vi "Add Core Dependencies.vi"(8 "error in (no error)":errorcluster, 11 "Item Ref in":T1 format="%.0x") -> (0 "error out":errorcluster, 3 "Device Ref out":T1 format="%.0x")   [LabVIEW 2017, in "DSF System Explorer.lvlib"]
uses:
  DSF System Explorer.lvlib
  <vilib>/NI Veristand/Custom Device API/Custom Device Item Ref.ctl
  <vilib>/NI Veristand/Custom Device API/Custom Device File Dependency.ctl
  <vilib>/NI Veristand/Custom Device API/Path Specification.ctl
  <vilib>/NI Veristand/Custom Device API/Path Type.ctl
  <vilib>/NI Veristand/Custom Device API/Custom Device Supported Target.ctl
  <vilib>/NI Veristand/Custom Device API/Custom Device API.lvlib
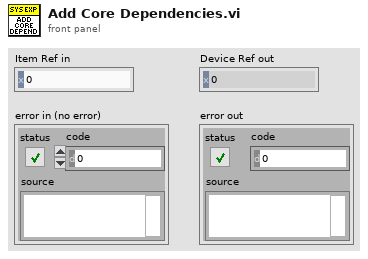
[diagram p1: front panel]
types:
  T1 = typedef "Custom Device API.lvlib/Custom Device Item Ref.ctl" = u64
  T2 = typedef "Custom Device API.lvlib/Custom Device Target Type.ctl" = enum16{"PharLap", "VxWorks", "Windows", "Linux_32_ARM", "Linux_x64"}
  T3 = typedef "Custom Device API.lvlib/Custom Device Supported Target.ctl" = enum16{"All", "PharLap", "VxWorks", "Windows", "Linux_32_ARM", "Linux_x64", "PharLap & Windows", "PharLap & VxWorks", "VxWorks & Windows"}
  T4 = typedef "Custom Device API.lvlib/Path Type.ctl" = enum16{"Absolute", "To Base", "To Common Data Dir", "To Application Data Dir"}
  T5 = typedef "Custom Device API.lvlib/Custom Device File Dependency.ctl" = cluster{"Source":T6, "RT Destination":path, "ForceDownload?":bool, "SupportedTarget":T3, "Version":string}
  T6 = typedef "Custom Device API.lvlib/Path Specification.ctl" = cluster{"Path":path, "Type":T4}
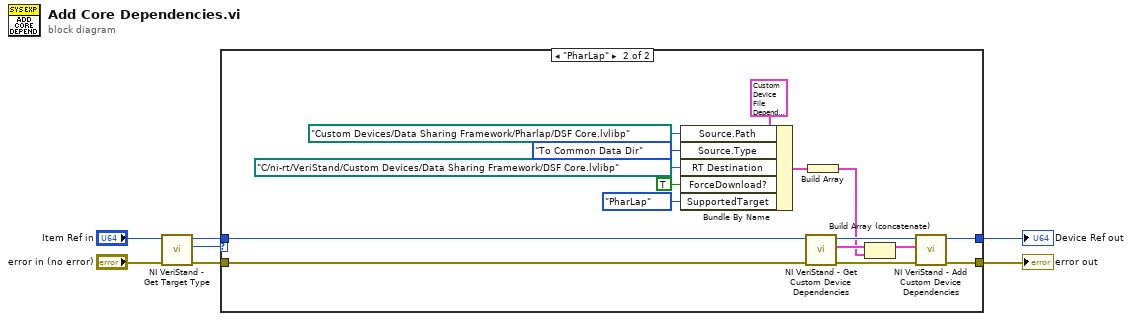
[diagram p0: block diagram]
diagram:
  n1 = call <vilib>:"NI VeriStand - Get Target Type.vi"("error in (no error)"="error in (no error)", "Item Ref in"="Item Ref in") -> ("error out"=w6:errorcluster, "Target Type"=w7:T2, "Item Ref out"=w5:T1)  [unwired: 7 in]
  n2 = case shown="\"PharLap\"" w7 {
    tunnel: [w9 w12] -> w1
    tunnel: [w8 w11] -> w2
    tunnel: w5 -> [w8 w13]
    tunnel: w6 -> [w9 w14]
    frame "Windows", Default {
      # "Don't add dependency for Windows or unsupported target type."
    }
    frame "PharLap" {
      n3 = Bundle By Name(cluster=T5 {"Source"={"Path"=path "", "Type"=enum."Absolute"}, "RT Destination"=path "", "ForceDownload?"=FALSE, "SupportedTarget"=enum."PharLap", "Version"=""} ("Dependencies"), "Source.Path"=path "Custom Devices/Data Sharing Framework/Pharlap/DSF Core.lvlibp", "Source.Type"=Path_Type."To Common Data Dir", "RT Destination"=path "C:/ni-rt/VeriStand/Custom Devices/Data Sharing Framework/DSF Core.lvlibp", "ForceDownload?"=TRUE, "SupportedTarget"=Custom_Device_Supported_Target."PharLap") -> (w19:T5)
      n4 = call <vilib>:"NI VeriStand - Get Custom Device Dependencies.vi"("error in (no error)"=w14, "Device Ref in"=w13) -> ("error out"=w17:errorcluster, "Dependencies"=w18:T5[], "Device Ref out"=w15:T1)  [unwired: 7 in]
      n5 = Build Array(w19) -> (w10:T5[])
      n6 = Build Array (concatenate)(w18, w10) -> (w16:T5[])
      n7 = call <vilib>:"NI VeriStand - Add Custom Device Dependencies.vi"("error in (no error)"=w17, "Dependencies"=w16, "Device Ref in"=w15) -> ("error out"=w12:errorcluster, "Device Ref out"=w11:T1)  [unwired: 7 in]
    }
  }
  "Device Ref out" <- w2
  "error out" <- w1
